vi "Motor Control final.vi"() -> ()   [LabVIEW 2017]
uses:
  Control 1.ctl
  Global 1.vi
  DynamixelSDK-3.7.31/labview/dxl_x86_c.lvlib/dxl_x86_c.lvlib
panel:
  in  "LA lower 0":bool
  in  "x":dbl
  in  "input variable":dbl=10.0
  in  "y":dbl=38.0
  in  "Y new 37":dbl
  in  "Meter":i32(knob) scale=0.0..800.0
  in  "Shot":bool
  out "Shot - Act/pas":bool
  out "motor 7":dbl
  out "dynamixel7_id":u8=1
  out "dynamixel6_id":u8=1
  out "motor 1 2":dbl
  out "motor 5":dbl
  out "motor 3 4":dbl
  in  "z value":dbl(slide) scale=32.0..52.0
  out "dynamixel5_id":u8=1
  out "dynamixel4_id":u8=1
  out "dynamixel3_id":T1=1
  out "dynamixel_error":string
  out "dynamixel_comm_result":string
  out "groupread_num":i32
  in  "LEN_PRO_\nPRESENT_POSITION":u16=4
  out "groupwrite_num":i32
  in  "LEN_PRO_\nGOAL_POSITION":u16=4
  in  "dynamixe2_id":u8=2
  in  "device_name":string="COM1"
  out "ADDR_PRO_\nPRESENT_POSITION":u16=611
  out "ADDR_PRO_\nGOAL_POSITION":u16=596
  out "ADDR_PRO_\nTORQUE_ENABLE":u16=562
  out "protocol_version":dbl=2.0
  in  "terminate":bool
  out "port_num":i32
  in  "dynamixel1_id":u8=1
  in  "baud_rate":i32=57600
  # "37~40(37)"
  # "0 or 1(0.7)"
  # "7 or 8(7)"
  # "7~11(10)"
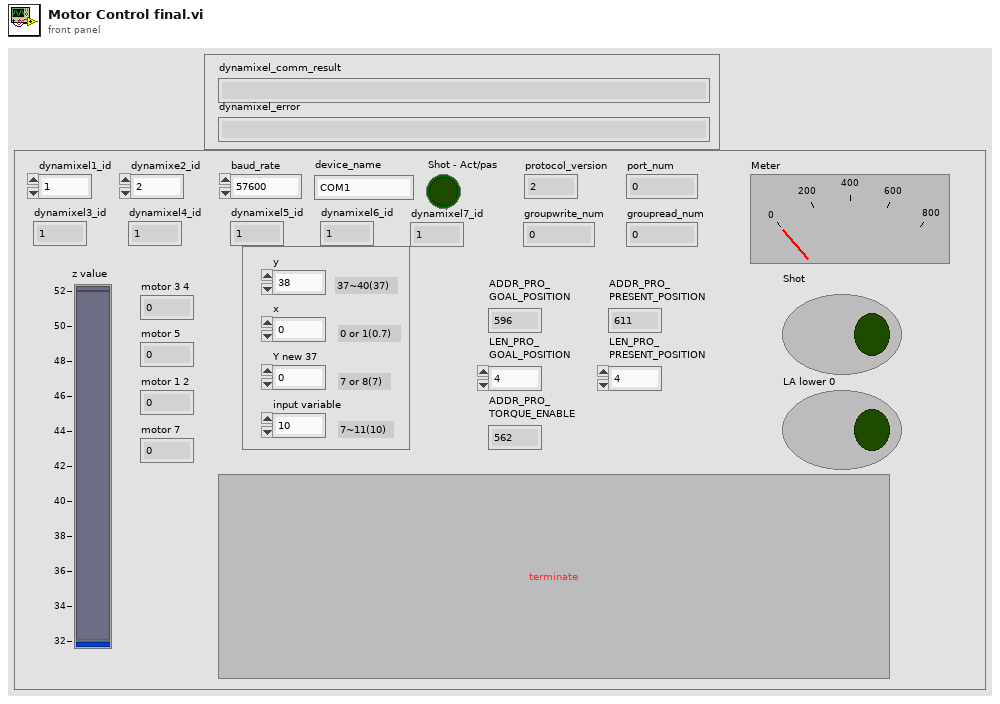
[diagram p1: front panel]
types:
  T1 = typedef "Control 1.ctl" = u8
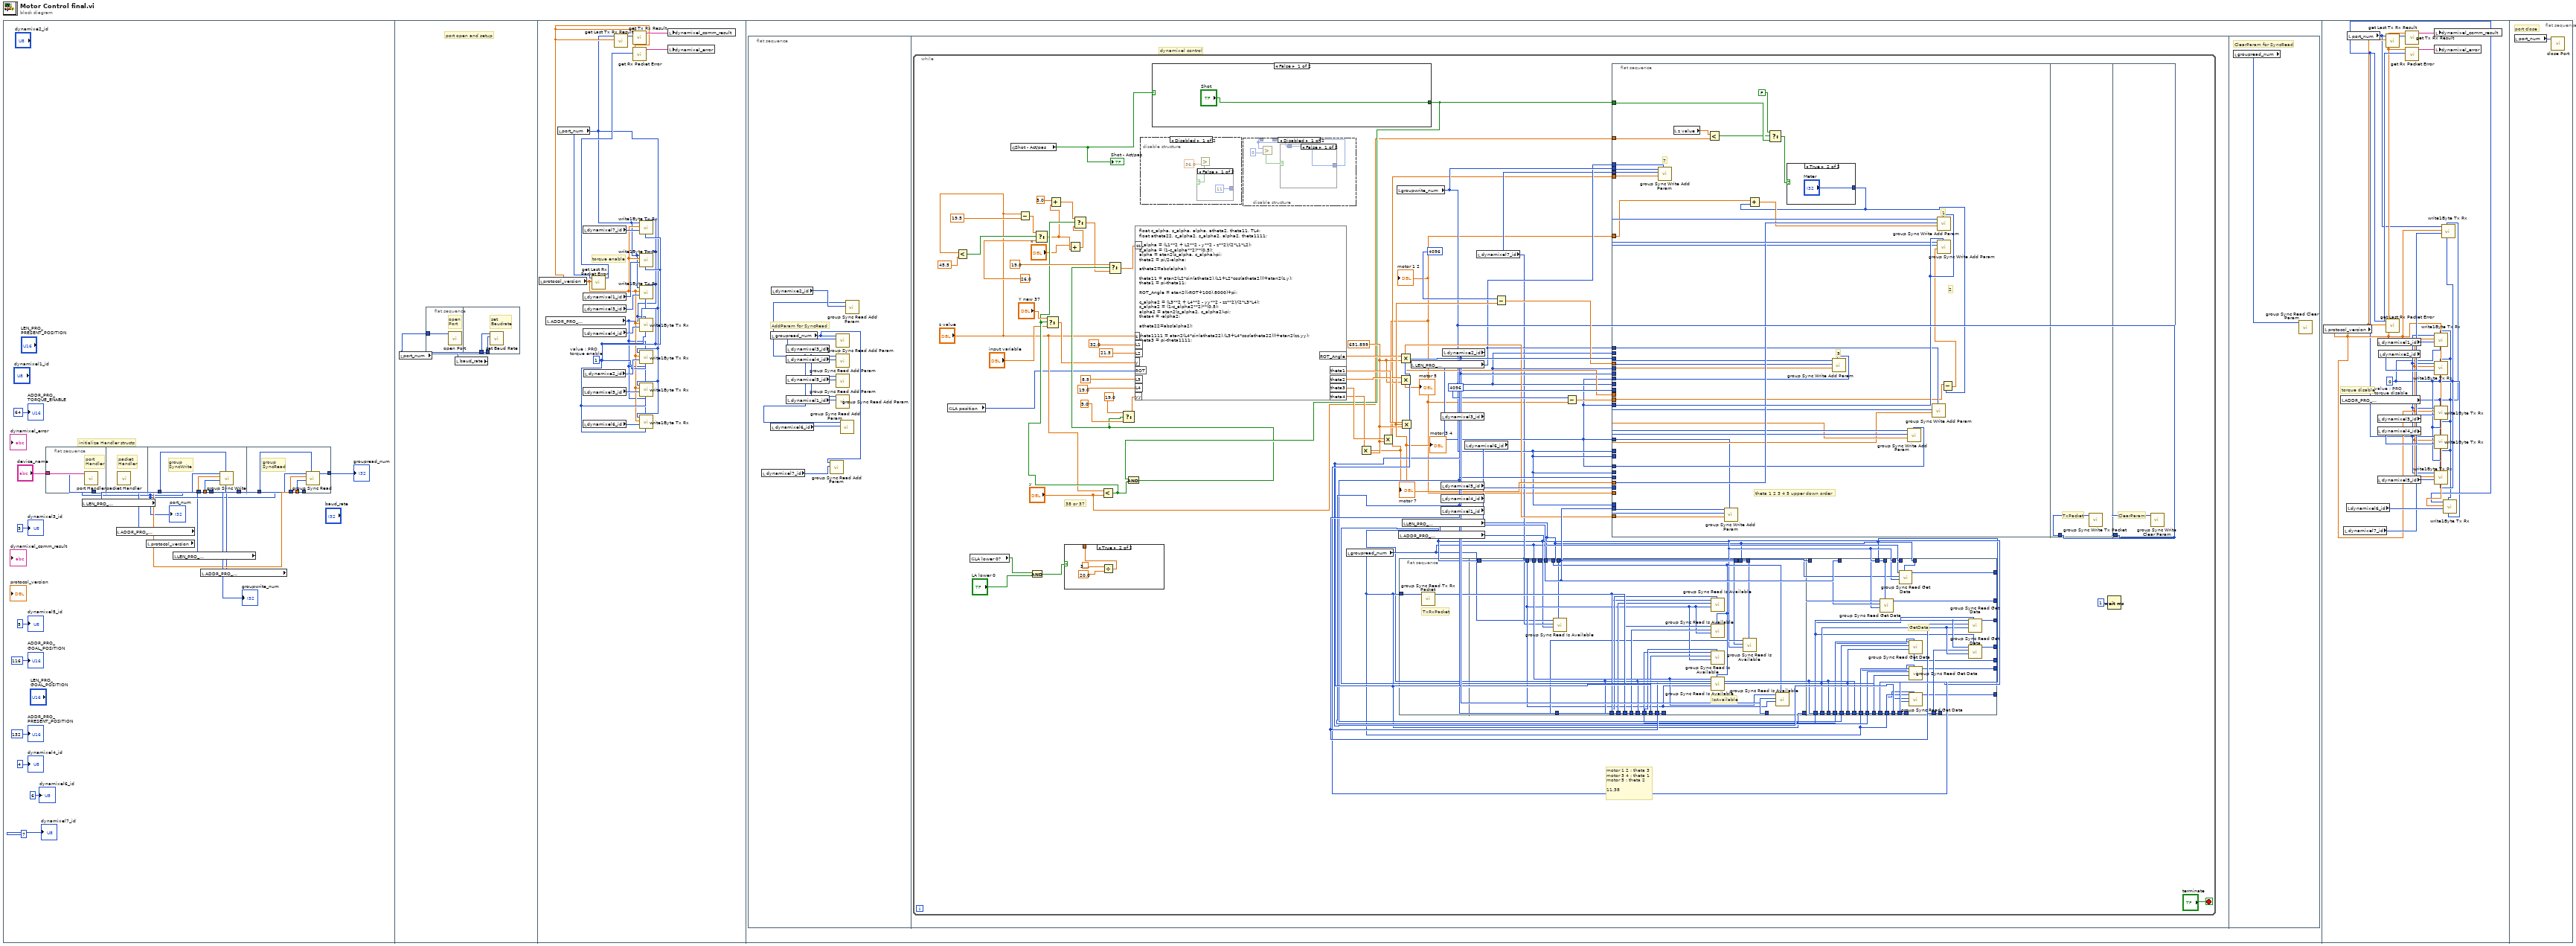
[diagram p0: block diagram]
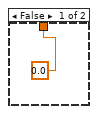
[diagram p2: hidden frame]
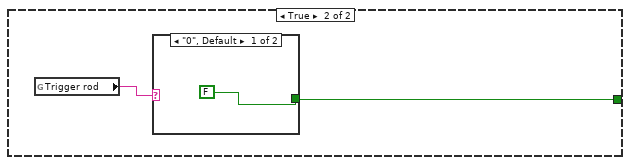
[diagram p3: hidden frame]
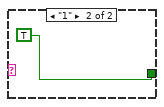
[diagram p4: hidden frame]
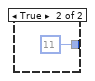
[diagram p5: hidden frame]
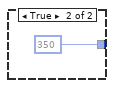
[diagram p7: hidden frame]
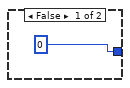
[diagram p9: hidden frame]
diagram:
  n1 = flat-sequence {
    frame #0 {
      # "initialize Handler structs"
      n2 = flat-sequence {
        tunnel: "device_name" -> [w19]
        tunnel: [w18] -> w10
        tunnel: w16 -> [w24]
        tunnel: w15 -> [w23]
        tunnel: w12 -> [w22]
        tunnel: w10 -> [w21]
        tunnel: [w20] -> w14
        tunnel: [w29] -> w13
        tunnel: w12 -> [w28]
        tunnel: w11 -> [w27]
        tunnel: w10 -> [w26]
        tunnel: w9 -> [w25]
        frame #0 {
          # "port\nHandler"
          n3 = call "port Handler.vi"("port_name"=w19) -> ("function return"=w18:i32)  [unwired: 10 in]
        }
        frame #1 {
          # "packet\nHandler"
          n4 = call "packet Handler.vi"() -> ()  [unwired: 12 in]
        }
        frame #2 {
          # "group\nSyncWrite"
          n5 = call "group Sync Write.vi"("data_length"=w24, "start_address"=w23, "protocol_version"=w22, "port_num"=w21) -> ("function return"=w20:i32)  [unwired: 7 in]
        }
        frame #3 {
          # "group\nSyncRead"
          n6 = call "group Sync Read.vi"("data_length"=w25, "start_address"=w27, "protocol_version"=w28, "port_num"=w26) -> ("function return"=w29:i32)  [unwired: 7 in]
        }
      }
      n7 = local read "LEN_PRO_\nGOAL_POSITION"() -> (w16:u16)
      n8 = local read "ADDR_PRO_\nGOAL_POSITION"() -> (w15:u16)
      n9 = local read "protocol_version"() -> (w12:dbl)
      n10 = local read "LEN_PRO_\nPRESENT_POSITION"() -> (w9:u16)
      n11 = local read "ADDR_PRO_\nPRESENT_POSITION"() -> (w11:u16)
      "port_num" <- w10
      "ADDR_PRO_\nTORQUE_ENABLE" <- u16 64 ("ADDR_PRO_\nTORQUE_ENABLE")
      "ADDR_PRO_\nGOAL_POSITION" <- u16 116 ("ADDR_PRO_\nGOAL_POSITION")
      "ADDR_PRO_\nPRESENT_POSITION" <- u16 132 ("ADDR_PRO_\nPRESENT_POSITION")
      "groupwrite_num" <- w14
      "groupread_num" <- w13
      "dynamixel3_id" <- T1 3 ("dynamixel3_id")
      "dynamixel4_id" <- u8 4 ("dynamixel4_id")
      "dynamixel5_id" <- u8 5 ("dynamixel5_id")
      "dynamixel6_id" <- u8 6 ("dynamixel6_id")
      "dynamixel7_id" <- u8 7 ("dynamixel7_id")
    }
    frame #1 {
      # "port open and setup"
      n12 = local read "port_num"() -> (w31:i32)
      n13 = flat-sequence {
        tunnel: w31 -> [w32]
        tunnel: w31 -> [w34]
        tunnel: w30 -> [w33]
        frame #0 {
          # "open\nPort"
          n14 = call "open Port.vi"("port_num"=w32) -> ()  [unwired: 10 in, 1 out]
        }
        frame #1 {
          # "set\nBaudrate"
          n15 = call "set Baud Rate.vi"("baudrate"=w33, "port_num"=w34) -> ()  [unwired: 9 in, 1 out]
        }
      }
      n16 = local read "baud_rate"() -> (w30:i32)
    }
    frame #2 {
      w38 = 1  # value : PRO torque enable
      # "torque enable"
      n17 = local read "protocol_version"() -> (w37:dbl)
      n18 = local read "ADDR_PRO_\nTORQUE_ENABLE"() -> (w35:u16)
      n19 = local read "port_num"() -> (w36:i32)
      n20 = local read "dynamixel7_id"() -> (w39:u8)
      n21 = local read "dynamixel1_id"() -> (w49:u8)
      n22 = local read "dynamixel3_id"() -> (w43:T1)
      n23 = local read "dynamixel4_id"() -> (w42:u8)
      n24 = local read "dynamixel5_id"() -> (w41:u8)
      n25 = local read "dynamixel6_id"() -> (w40:u8)
      n26 = local read "dynamixe2_id"() -> (w48:u8)
      n27 = call "get Last Rx Packet Error.vi"("protocol_version"=w37, "port_num"=w36) -> ("function return"=w46:u8)  [unwired: 9 in]
      n28 = call "get Last Tx Rx Result.vi"("protocol_version"=w37, "port_num"=w36) -> ("function return"=w47:i32)  [unwired: 9 in]
      n29 = call "get Tx Rx Result.vi"("result"=w47, "protocol_version"=w37) -> ("function return"=w45:string)  [unwired: 9 in]
      n30 = call "get Rx Packet Error.vi"("error"=w46, "protocol_version"=w37) -> ("function return"=w44:string)  [unwired: 9 in]
      n31 = call "write1Byte Tx Rx.vi"("data"=w38, "address"=w35, "id"=w39, "protocol_version"=w37, "port_num"=w36) -> ()  [unwired: 7 in]
      n32 = call "write1Byte Tx Rx.vi"("data"=w38, "address"=w35, "id"=w49, "protocol_version"=w37, "port_num"=w36) -> ()  [unwired: 7 in]
      n33 = call "write1Byte Tx Rx.vi"("data"=w38, "address"=w35, "id"=w43, "protocol_version"=w37, "port_num"=w36) -> ()  [unwired: 7 in]
      n34 = call "write1Byte Tx Rx.vi"("data"=w38, "address"=w35, "id"=w42, "protocol_version"=w37, "port_num"=w36) -> ()  [unwired: 7 in]
      n35 = call "write1Byte Tx Rx.vi"("data"=w38, "address"=w35, "id"=w48, "protocol_version"=w37, "port_num"=w36) -> ()  [unwired: 7 in]
      n36 = call "write1Byte Tx Rx.vi"("data"=w38, "address"=w35, "id"=w41, "protocol_version"=w37, "port_num"=w36) -> ()  [unwired: 7 in]
      n37 = call "write1Byte Tx Rx.vi"("data"=w38, "address"=w35, "id"=w40, "protocol_version"=w37, "port_num"=w36) -> ()  [unwired: 7 in]
      n38 = local write "dynamixel_comm_result"(w45) -> ()
      n39 = local write "dynamixel_error"(w44) -> ()
    }
    frame #3 {
      n40 = flat-sequence {
        frame #0 {
          # "AddParam for SyncRead"
          n41 = local read "dynamixel7_id"() -> (w51:u8)
          n42 = local read "groupread_num"() -> (w50:i32)
          n43 = local read "dynamixel6_id"() -> (w52:u8)
          n44 = local read "dynamixe2_id"() -> (w56:u8)
          n45 = local read "dynamixel3_id"() -> (w55:T1)
          n46 = local read "dynamixel4_id"() -> (w54:u8)
          n47 = local read "dynamixel5_id"() -> (w53:u8)
          n48 = local read "dynamixel1_id"() -> (w57:u8)
          n49 = call "group Sync Read Add Param.vi"("id"=w51, "group_num"=w50) -> ()  [unwired: 9 in, 1 out]
          n50 = call "group Sync Read Add Param.vi"("id"=w55, "group_num"=w50) -> ()  [unwired: 9 in, 1 out]
          n51 = call "group Sync Read Add Param.vi"("id"=w54, "group_num"=w50) -> ()  [unwired: 9 in, 1 out]
          n52 = call "group Sync Read Add Param.vi"("id"=w53, "group_num"=w50) -> ()  [unwired: 9 in, 1 out]
          n53 = call "group Sync Read Add Param.vi"("id"=w57, "group_num"=w50) -> ()  [unwired: 9 in, 1 out]
          n54 = call "group Sync Read Add Param.vi"("id"=w52, "group_num"=w50) -> ()  [unwired: 9 in, 1 out]
          n55 = call "group Sync Read Add Param.vi"("id"=w56, "group_num"=w50) -> ()  [unwired: 9 in, 1 out]
        }
        frame #1 {
          # "dynamixel control"
          n56 = while {
            stop <- "terminate" stop-if-true
            w91 = 651.899
            # "38 or 37"
            # "motor 1 2 : theta 3\nmotor 3 4 : theta 1\nmotor 5 : theta 2\n\n11.38"
            n57 = global read "Global 1.vi" "LA position"() -> (w58:i32)
            n58 = Less?(x="z value", y=45.5) -> (x < y?=w87:bool)
            n59 = global read "Global 1.vi" "LA lower 0?"() -> (w61:bool)
            n60 = global read "Global 1.vi" "Shot - Act/pas"() -> (w84:bool)
            "Shot - Act/pas" <- w84
            n61 = Subtract(x="z value", y=19.5 ("t")) -> (x-y=w82:dbl)
            n62 = And(x=w61, y="LA lower 0") -> (x .and. y?=w62:bool)
            n63 = Select(t=w82, s=w87, f=26.0) -> (s? t:f=w66:dbl)
            n64 = Add(x=3.0, y=w66) -> (x+y=w70:dbl)
            n65 = case shown="True" w62 {
              tunnel: [0.0 w121] -> _
              frame False {
              }
              frame True {
                n66 = Divide(x=3.141592653589793, y=20.0) -> (x/y=w121:dbl)
              }
            }
            n67 = Add(x="x", y=w66) -> (x+y=w64:dbl)
            n68 = Less?(x="z value", y="y") -> (x < y?=w72:bool)
            n69 = Select(t="Y new 37", s=w72, f="input variable") -> (s? t:f=w73:dbl)
            n70 = Select(t=w70, s=w72, f=w64) -> (s? t:f=w69:dbl)
            n71 = disable-structure shown="Disabled" {
              frame Disabled {
                n72 = Greater?(y=36.0) -> (x=w131:dbl, 0:w129:bool)
                n73 = case shown="False" w129 {
                  tunnel: [11 11] -> _
                  frame False {
                  }
                  frame True {
                  }
                }
              }
              frame Enabled {
              }
            }
            n74 = case shown="False" w84 {
              tunnel: ["Shot" w125] -> w78
              frame False {
              }
              frame True {
                n75 = global read "Global 1.vi" "Trigger rod"() -> (w126:string)
                n76 = case shown="\"0\", Default" w126 {
                  tunnel: [FALSE TRUE] -> w125
                  frame "0", Default {
                  }
                  frame "1" {
                  }
                }
              }
            }
            n77 = And(x=w78, y=w72) -> (x .and. y?=w76:bool)
            n78 = Select(t=19.0, s=w76, f=w69) -> (s? t:f=w75:dbl)
            n79 = Select(t=19.0, s=w76, f=5.0 ("input variable")) -> (s? t:f=w79:dbl)
            n80 = formula code="float c_alpha, s_alpha, alpha, atheta2, theta11, TL4;\nfloat atheta22, c_alpha2, s_alpha2, alpha2, theta1111;\n\nc_alpha = (L1**2 + L2**2 - y**2 - z**2)/(2*L1*L2);\ns_alpha = (1-c_alpha**2)**(0.5);\nalpha = atan2(s_alpha, c_alpha)-pi;\ntheta2 = pi/2-alpha;\n\natheta2=abs(alpha);\n\ntheta11 = atan2(L2*sin(atheta2),(L1+L2*cos(atheta2)))+atan2(z,y);\ntheta1 = pi-theta11;\n\nROT_Angle = atan2((-ROT+100),8000)+pi;\n\nc_alpha2 = (L3**2 + L4**2 - yy**2 - zz**2)/(2*L3*L4);\ns_alpha2 = (1-c_alpha2**2)**(0.5);\nalpha2 = atan2(s_alpha2, c_alpha2)-pi;\ntheta4 = -alpha2;\n\natheta22=abs(alpha2);\n\ntheta1111 = atan2(L4*sin(atheta22),(L3+L4*cos(atheta22)))+atan2(zz,yy);\ntheta3 = pi-theta1111;"("z"="z value", "L1"=32.0 ("input variable"), "L2"=21.5 ("input variable"), "y"=w73, "ROT"=w58, "L3"=8.5 ("input variable"), "L4"=19.0 ("input variable"), "yy"=w79, "zz"=w75) -> ("theta1"=w110:dbl, "theta2"=w109:dbl, "theta3"=w111:dbl, "ROT_Angle"=w100:dbl, "theta4"=w92:dbl)
            n81 = disable-structure shown="Disabled" {
              disable-tunnel: [w135 _] -> _
              disable-tunnel: _ -> [w134 _]
              frame Disabled {
                n82 = Greater?(x=w134, y=0) -> (0:w136:bool)
                n83 = case shown="False" w136 {
                  tunnel: [w138 350] -> w135
                  tunnel: w134 -> [w138 _]
                  frame False {
                  }
                  frame True {
                  }
                }
              }
              frame Enabled {
              }
            }
            n84 = local read "groupread_num"() -> (w95:i32)
            n85 = Multiply(x=w92, y=w91) -> (x*y=w90:dbl)
            "motor 7" <- w90
            n86 = Multiply(x=w111, y=w91) -> (x*y=w85:dbl)
            "motor 1 2" <- w85
            n87 = local read "groupwrite_num"() -> (w99:i32)
            n88 = local read "ADDR_PRO_\nPRESENT_POSITION"() -> (w96:u16)
            n89 = Multiply(x=w100, y=w91) -> (x*y=w101:dbl)
            n90 = Multiply(x=w109, y=w91) -> (x*y=w103:dbl)
            "motor 5" <- w103
            n91 = flat-sequence {
              tunnel: w95 -> [w140]
              tunnel: w95 -> [w161]
              tunnel: w118 -> [w160]
              tunnel: w117 -> [w159]
              tunnel: w94 -> [w158]
              tunnel: w94 -> [w157]
              tunnel: w94 -> [w156]
              tunnel: w95 -> [w155]
              tunnel: w95 -> [w154]
              tunnel: w95 -> [w153]
              tunnel: w116 -> [w152]
              tunnel: w115 -> [w151]
              tunnel: w114 -> [w150]
              tunnel: w96 -> [w149]
              tunnel: w95 -> [w148]
              tunnel: w102 -> [w147]
              tunnel: w96 -> [w146]
              tunnel: w94 -> [w145]
              tunnel: w97 -> [w144]
              tunnel: w94 -> [w143]
              tunnel: w95 -> [w142]
              tunnel: w96 -> [w141]
              tunnel: w95 -> [w193]
              tunnel: w118 -> [w192]
              tunnel: w117 -> [w188]
              tunnel: w96 -> [w189]
              tunnel: w94 -> [w187]
              tunnel: [w191] -> _
              tunnel: [w190] -> _
              tunnel: w95 -> [w186]
              tunnel: w95 -> [w185]
              tunnel: w95 -> [w184]
              tunnel: w116 -> [w183]
              tunnel: w115 -> [w182]
              tunnel: w114 -> [w181]
              tunnel: w96 -> [w180]
              tunnel: w96 -> [w179]
              tunnel: w96 -> [w178]
              tunnel: w94 -> [w177]
              tunnel: w94 -> [w176]
              tunnel: w94 -> [w175]
              tunnel: [w174] -> _
              tunnel: [w173] -> _
              tunnel: [w172] -> _
              tunnel: w95 -> [w171]
              tunnel: w102 -> [w170]
              tunnel: w96 -> [w169]
              tunnel: w94 -> [w168]
              tunnel: [w167] -> _
              tunnel: w97 -> [w166]
              tunnel: w96 -> [w165]
              tunnel: w95 -> [w164]
              tunnel: w94 -> [w163]
              tunnel: [w162] -> _
              frame #0 {
                # "TxRxPacket"
                n92 = call "group Sync Read Tx Rx Packet.vi"("group_num"=w140) -> ()  [unwired: 11 in]
              }
              frame #1 {
                # "IsAvailable"
                n93 = call "group Sync Read Is Available.vi"("data_length"=w143, "address"=w141, "id"=w144, "group_num"=w142) -> ()  [unwired: 7 in, 1 out]
                n94 = call "group Sync Read Is Available.vi"("data_length"=w156, "address"=w149, "id"=w150, "group_num"=w153) -> ()  [unwired: 7 in, 1 out]
                n95 = call "group Sync Read Is Available.vi"("data_length"=w157, "address"=w149, "id"=w151, "group_num"=w154) -> ()  [unwired: 7 in, 1 out]
                n96 = call "group Sync Read Is Available.vi"("data_length"=w158, "address"=w149, "id"=w152, "group_num"=w155) -> ()  [unwired: 7 in, 1 out]
                n97 = call "group Sync Read Is Available.vi"("data_length"=w157, "address"=w149, "id"=w160, "group_num"=w161) -> ()  [unwired: 7 in, 1 out]
                n98 = call "group Sync Read Is Available.vi"("data_length"=w145, "address"=w146, "id"=w147, "group_num"=w148) -> ()  [unwired: 7 in, 1 out]
                n99 = call "group Sync Read Is Available.vi"("data_length"=w157, "address"=w149, "id"=w159, "group_num"=w161) -> ()  [unwired: 7 in, 1 out]
              }
              frame #2 {
                # "GetData"
                n100 = call "group Sync Read Get Data.vi"("data_length"=w168, "address"=w169, "id"=w170, "group_num"=w171) -> ("function return"=w167:u32)  [unwired: 7 in]
                n101 = call "group Sync Read Get Data.vi"("data_length"=w163, "address"=w165, "id"=w166, "group_num"=w164) -> ("function return"=w162:u32)  [unwired: 7 in]
                n102 = call "group Sync Read Get Data.vi"("data_length"=w175, "address"=w178, "id"=w181, "group_num"=w184) -> ("function return"=w172:u32)  [unwired: 7 in]
                n103 = call "group Sync Read Get Data.vi"("data_length"=w176, "address"=w179, "id"=w182, "group_num"=w185) -> ("function return"=w173:u32)  [unwired: 7 in]
                n104 = call "group Sync Read Get Data.vi"("data_length"=w177, "address"=w180, "id"=w183, "group_num"=w186) -> ("function return"=w174:u32)  [unwired: 7 in]
                n105 = call "group Sync Read Get Data.vi"("data_length"=w187, "address"=w189, "id"=w192, "group_num"=w193) -> ("function return"=w191:u32)  [unwired: 7 in]
                n106 = call "group Sync Read Get Data.vi"("data_length"=w187, "address"=w189, "id"=w188, "group_num"=w193) -> ("function return"=w190:u32)  [unwired: 7 in]
              }
            }
            n107 = Multiply(x=w110, y=w91) -> (x*y=w104:dbl)
            "motor 3 4" <- w104
            n108 = local read "LEN_PRO_\nPRESENT_POSITION"() -> (w94:u16)
            n109 = local read "LEN_PRO_\nGOAL_POSITION"() -> (w98:u16)
            n110 = local read "dynamixel3_id"() -> (w116:T1)
            n111 = local read "dynamixel5_id"() -> (w114:u8)
            n112 = local read "dynamixel4_id"() -> (w115:u8)
            n113 = local read "dynamixel1_id"() -> (w118:u8)
            n114 = local read "dynamixe2_id"() -> (w117:u8)
            n115 = local read "dynamixel6_id"() -> (w102:u8)
            n116 = local read "dynamixel7_id"() -> (w97:u8)
            n117 = Subtract(x=4096, y=w104) -> (x-y=w105:dbl)
            n118 = Subtract(x=4096, y=w85) -> (x-y=w106:dbl)
            n119 = flat-sequence {
              tunnel: w98 -> [w229]
              tunnel: w99 -> [w228]
              tunnel: w99 -> [w227]
              tunnel: w118 -> [w226]
              tunnel: w117 -> [w225]
              tunnel: w99 -> [_]
              tunnel: w99 -> [w224]
              tunnel: w99 -> [w223]
              tunnel: w99 -> [w222]
              tunnel: w98 -> [w221]
              tunnel: w98 -> [w220]
              tunnel: w98 -> [w209]
              tunnel: w116 -> [w219]
              tunnel: w115 -> [w218]
              tunnel: w114 -> [w217]
              tunnel: w106 -> [w202]
              tunnel: w85 -> [_]
              tunnel: w105 -> [w214]
              tunnel: w104 -> [w215]
              tunnel: w103 -> [w216]
              tunnel: w102 -> [w213]
              tunnel: w99 -> [w212]
              tunnel: w98 -> [w211]
              tunnel: w101 -> [w210]
              tunnel: w97 -> [w208]
              tunnel: w99 -> [w207]
              tunnel: w98 -> [w206]
              tunnel: w90 -> [w205]
              tunnel: w85 -> [w204]
              tunnel: w78 -> [w198]
              tunnel: "y" -> [w194]
              tunnel: w99 -> [w232]
              tunnel: w99 -> [w233]
              frame #0 {
                # "5"
                # "2"
                # "1"
                # "7"
                # "theta 1 2 3 4 5 upper down order"
                n120 = call "group Sync Write Add Param.vi"("data_length"=w206, "data"=w205, "id"=w208, "group_num"=w207) -> ()  [unwired: 7 in, 1 out]
                n121 = local read "z value"() -> (w199:dbl)
                n122 = Less?(x=w199, y=w194) -> (x < y?=w195:bool)
                n123 = call "group Sync Write Add Param.vi"("data_length"=w211, "data"=w210, "id"=w213, "group_num"=w212) -> ()  [unwired: 7 in, 1 out]
                n124 = Select(t=FALSE, s=w195, f=w198) -> (s? t:f=w197:bool)
                n125 = case shown="True" w197 {
                  tunnel: [0 "Meter"] -> w201
                  frame False {
                  }
                  frame True {
                  }
                }
                n126 = Add(x=w204, y=w201) -> (x+y=w203:dbl)
                n127 = call "group Sync Write Add Param.vi"("data_length"=w209, "data"=w216, "id"=w217, "group_num"=w224) -> ()  [unwired: 7 in, 1 out]
                n128 = call "group Sync Write Add Param.vi"("data_length"=w220, "data"=w215, "id"=w218, "group_num"=w223) -> ()  [unwired: 7 in, 1 out]
                n129 = call "group Sync Write Add Param.vi"("data_length"=w221, "data"=w214, "id"=w219, "group_num"=w222) -> ()  [unwired: 7 in, 1 out]
                n130 = call "group Sync Write Add Param.vi"("data_length"=w229, "data"=w203, "id"=w226, "group_num"=w228) -> ()  [unwired: 7 in, 1 out]
                n131 = Subtract(x=w202, y=w201) -> (x-y=w200:dbl)
                n132 = call "group Sync Write Add Param.vi"("data_length"=w229, "data"=w200, "id"=w225, "group_num"=w227) -> ()  [unwired: 7 in, 1 out]
              }
              frame #1 {
                # "TxPacket"
                n133 = call "group Sync Write Tx Packet.vi"("group_num"=w232) -> ()  [unwired: 11 in]
              }
              frame #2 {
                # "ClearParam"
                n134 = call "group Sync Write Clear Param.vi"("group_num"=w233) -> ()  [unwired: 11 in]
              }
            }
            n135 = Wait (ms)(milliseconds to wait=u32 1) -> ()  [unwired: 1 out]
          }
        }
        frame #2 {
          # "ClearParam for SyncRead"
          n136 = local read "groupread_num"() -> (w234:i32)
          n137 = call "group Sync Read Clear Param.vi"("group_num"=w234) -> ()  [unwired: 11 in]
        }
      }
    }
    frame #4 {
      w236 = 0  # value : PRO torque disable
      # "torque disable"
      n138 = local read "protocol_version"() -> (w238:dbl)
      n139 = local read "ADDR_PRO_\nTORQUE_ENABLE"() -> (w235:u16)
      n140 = local read "dynamixel7_id"() -> (w239:u8)
      n141 = local read "dynamixel6_id"() -> (w240:u8)
      n142 = local read "port_num"() -> (w237:i32)
      n143 = local read "dynamixel1_id"() -> (w249:u8)
      n144 = local read "dynamixel3_id"() -> (w243:T1)
      n145 = local read "dynamixel4_id"() -> (w241:u8)
      n146 = local read "dynamixel5_id"() -> (w242:u8)
      n147 = local read "dynamixe2_id"() -> (w248:u8)
      n148 = call "get Last Tx Rx Result.vi"("protocol_version"=w238, "port_num"=w237) -> ("function return"=w246:i32)  [unwired: 9 in]
      n149 = call "get Last Rx Packet Error.vi"("protocol_version"=w238, "port_num"=w237) -> ("function return"=w247:u8)  [unwired: 9 in]
      n150 = call "get Tx Rx Result.vi"("result"=w246, "protocol_version"=w238) -> ("function return"=w245:string)  [unwired: 9 in]
      n151 = call "get Rx Packet Error.vi"("error"=w247, "protocol_version"=w238) -> ("function return"=w244:string)  [unwired: 9 in]
      n152 = local write "dynamixel_comm_result"(w245) -> ()
      n153 = local write "dynamixel_error"(w244) -> ()
      n154 = call "write1Byte Tx Rx.vi"("data"=w236, "address"=w235, "id"=w249, "protocol_version"=w238, "port_num"=w237) -> ()  [unwired: 7 in]
      n155 = call "write1Byte Tx Rx.vi"("data"=w236, "address"=w235, "id"=w248, "protocol_version"=w238, "port_num"=w237) -> ()  [unwired: 7 in]
      n156 = call "write1Byte Tx Rx.vi"("data"=w236, "address"=w235, "id"=w243, "protocol_version"=w238, "port_num"=w237) -> ()  [unwired: 7 in]
      n157 = call "write1Byte Tx Rx.vi"("data"=w236, "address"=w235, "id"=w241, "protocol_version"=w238, "port_num"=w237) -> ()  [unwired: 7 in]
      n158 = call "write1Byte Tx Rx.vi"("data"=w236, "address"=w235, "id"=w242, "protocol_version"=w238, "port_num"=w237) -> ()  [unwired: 7 in]
      n159 = call "write1Byte Tx Rx.vi"("data"=w236, "address"=w235, "id"=w239, "protocol_version"=w238, "port_num"=w237) -> ()  [unwired: 7 in]
      n160 = call "write1Byte Tx Rx.vi"("data"=w236, "address"=w235, "id"=w240, "protocol_version"=w238, "port_num"=w237) -> ()  [unwired: 7 in]
    }
    frame #5 {
      # "port close"
      n161 = local read "port_num"() -> (w250:i32)
      n162 = call "close Port.vi"("port_num"=w250) -> ()  [unwired: 11 in]
    }
  }
